vi "Stop Core.vi"(10 "final error code":i32, 11 "MuxActor in":refnum<class "MuxActor.lvclass">) -> (3 "MuxActor out":refnum<class "MuxActor.lvclass">)   [LabVIEW 2022 SP3, in "VideoMux.lvlib" / "MuxActor.lvclass"]
doc: "(<B>Filename</B>: Actor Framework.lvlib:Actor.lvclass:Stop Core.vi)\n\nDefines what the actor does before it stops. Use the <B>final error code</B> input to determine whether the actor shut down in response to an error.\n\nBy default, this method does nothing. A descendant class may override it to define behavior, such as shutting down any processes the actor initiated in its override of the Actor Core method."
uses:
  MuxActor.lvclass
  MuxActor.lvclass/MuxActor.ctl
  <vilib>/ActorFramework/Actor/Actor.lvclass
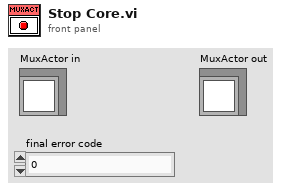
[diagram p1: front panel]
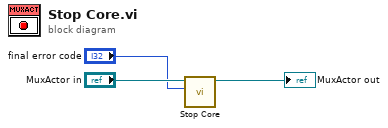
[diagram p0: block diagram]
diagram:
  n1 = call-parent "Stop Core.vi"("final error code"="final error code", "Actor in"="MuxActor in") -> ("Actor out"=→"MuxActor out":refnum<class "MuxActor.lvclass">)  [unwired: 9 in]
